vi "Find Paths in Map Relative to LV Root.vi"(11 "Code Coverage":map{path, dbl}(c390)) -> (3 "Array":path[](array[path]))   [LabVIEW 2020, in "LUnit Tests.lvlib" / "Coverage Test.lvclass"]
uses:
  Coverage Test.lvclass
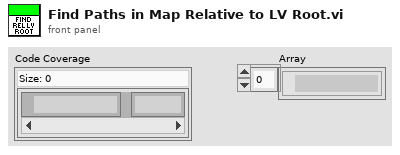
[diagram p1: front panel]
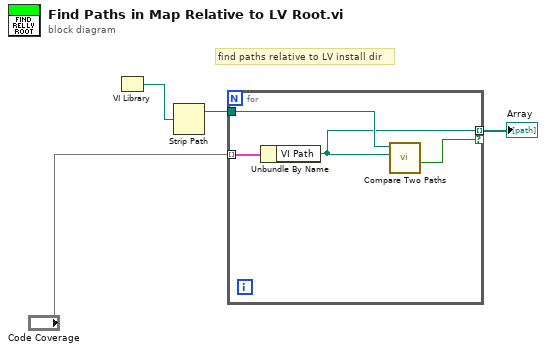
[diagram p0: block diagram]
diagram:
  # "find paths relative to LV install dir"
  n1 = VI Library() -> (path=w1:path)
  n2 = Strip Path(path=w1) -> (stripped path=w2:path)  [unwired: 1 out]
  n3 = for {
    tunnel: "Code Coverage" -> [w8] mode=indexing
    tunnel: w2 -> [w7]
    tunnel: [w6] -> w3 mode=indexing if=w5
    n4 = Unbundle By Name(w8) -> ("VI Path"=w6:path)
    n5 = call <vilib>:"Compare Two Paths.vi"("Path 2"=w6, "Path 1"=w7) -> ("Path 2 Relative to Path 1?"=w5:bool)  [unwired: 6 in, 3 out]
  }
  "Array" <- w3
